vi "与工控机交互(子VI).vi"   [LabVIEW 2016, in "数据传输系统.lvlib"]
uses:
  <vilib>/ptbypt/NI_PtbyPt.lvlib
types:
  T1 = cluster{"setini":string, "sysini":string, "hechaini":string, "actualwrite":string, "actualread":string, "datasent":string, "反控命令信息队列":string, "反控与仪器交互":string}
  T2 = cluster{"仪器状态":u16[], "试剂余量":u16[], "各参数测量间隔":u16[], "关键参数":u16[], "校准点信息":u16[], "告警信息":u16[], "系统信息":u16[]}
  T3 = cluster{"[0]":bool, "[1]":bool, "[2]":bool, "[3]":bool, "[4]":bool}
  T4 = cluster{"[0]":bool, "[1]":bool, "[2]":bool, "[3]":bool, "[4]":bool, "[5]":bool}
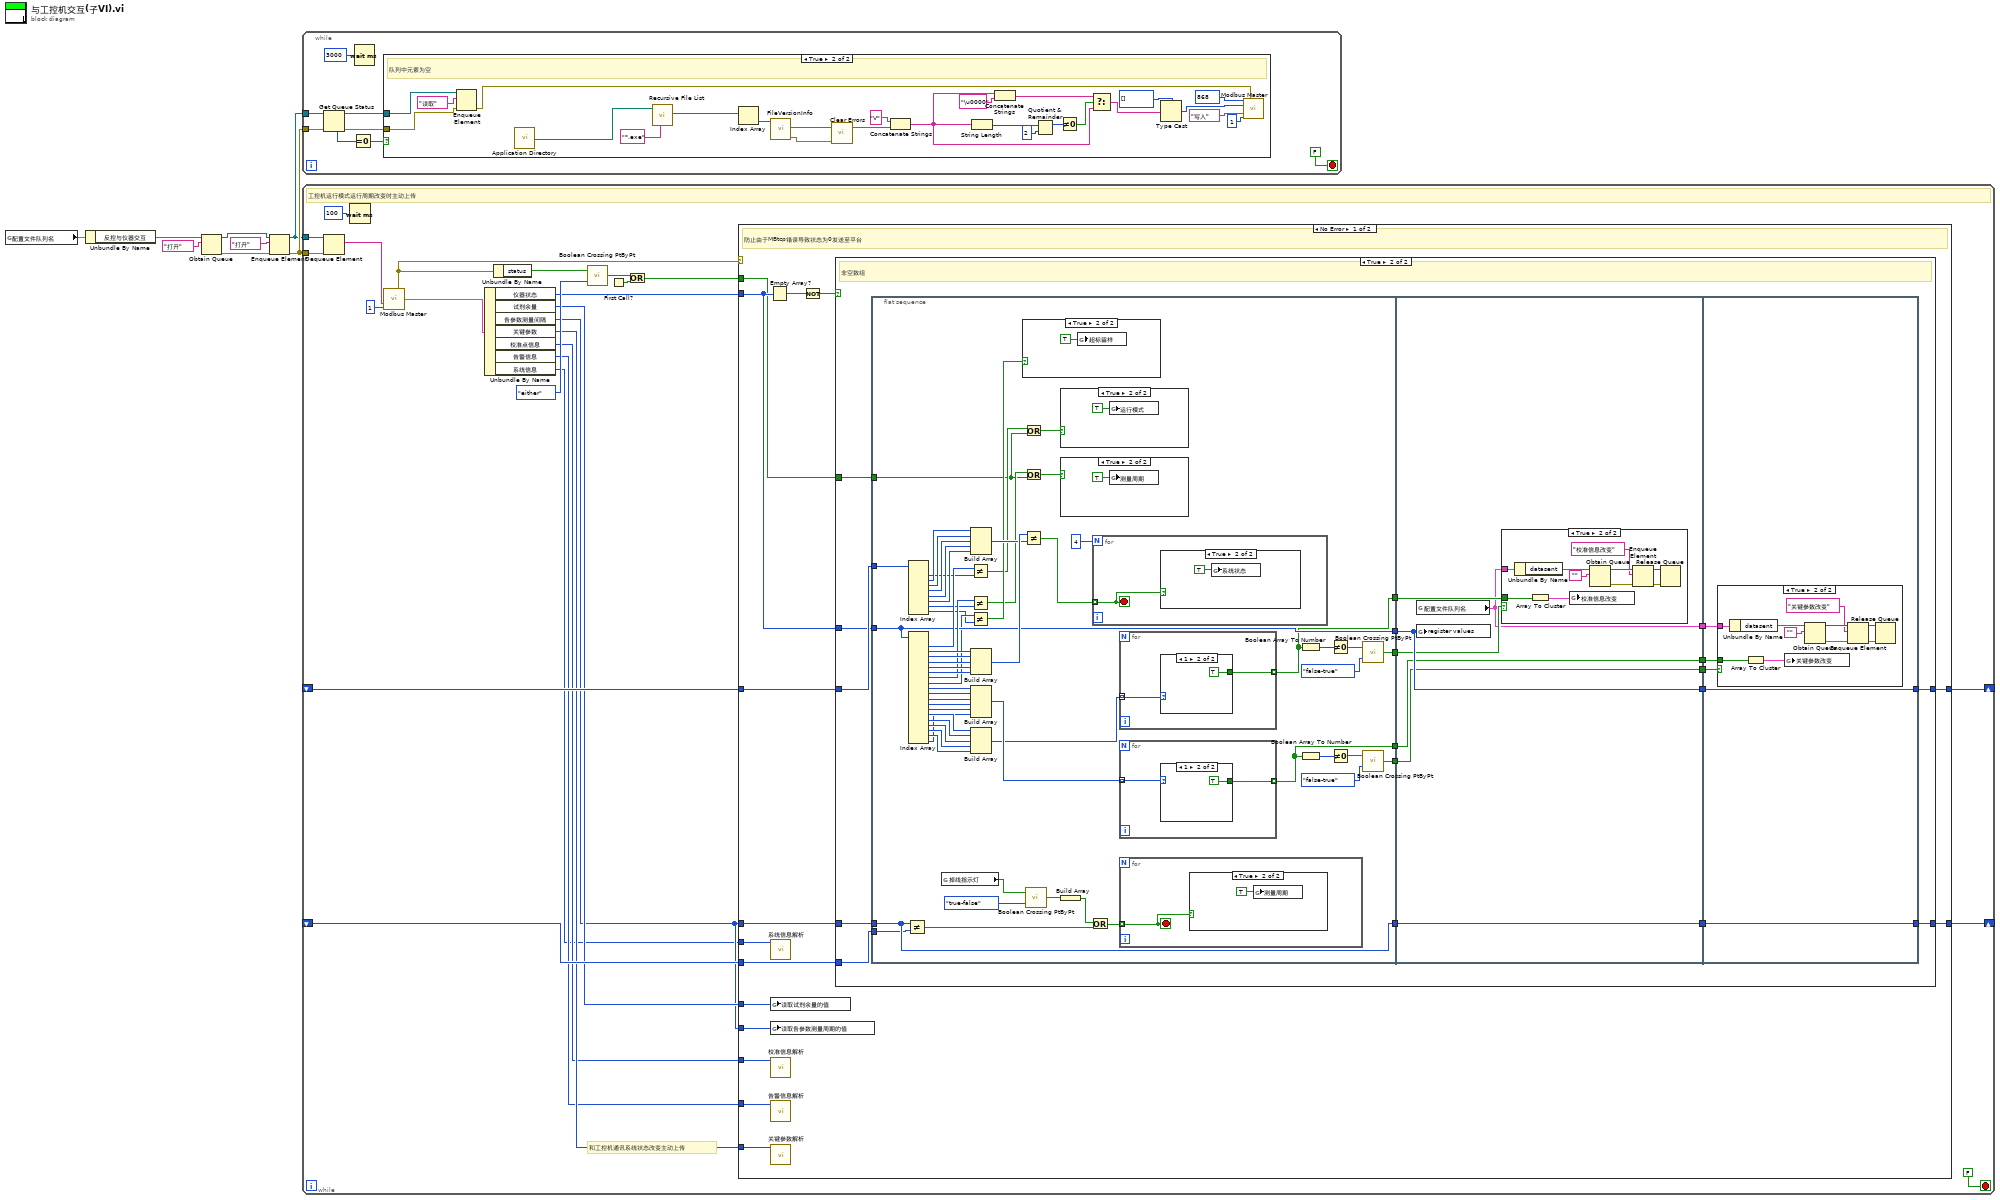
[diagram p0: block diagram]
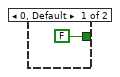
[diagram p4: hidden frame]
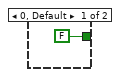
[diagram p5: hidden frame]
diagram:
  n1 = global read "全局1.vi" "配置文件队列名"() -> (w1:T1)
  n2 = Unbundle By Name(w1) -> ("反控与仪器交互"=w2:string)
  n3 = Obtain Queue(name (unnamed)=w2, element data type="打开" ("读取写入选择")) -> (queue out=w4:refnum<queue>, error out=w5:errorcluster)  [unwired: 3 in, 1 out]
  n4 = Enqueue Element(queue=w4, element="打开" ("读取写入选择"), error in (no error)=w5) -> (queue out=w6:refnum<queue>, error out=w7:errorcluster)  [unwired: 1 in, 1 out]
  n5 = while {
    tunnel: w6 -> [w13]
    tunnel: w7 -> [w12]
    stop <- FALSE stop-if-true
    n6 = Get Queue Status(queue=w13, error in (no error)=w12) -> (queue out=w10:refnum<queue>, error out=w9:errorcluster, # elements in queue=w14:i32)  [unwired: 1 in, 5 out]
    n7 = Equal To 0?(x=w14) -> (x = 0?=w11:bool)
    n8 = Wait (ms)(milliseconds to wait=u32 3000 ("等待时间（毫秒）")) -> ()  [unwired: 1 out]
    n9 = case shown="True" w11 {
      tunnel: w10 -> [_ w39]
      tunnel: w9 -> [_ w38]
      frame False {
      }
      frame True {
        # "队列中元素为空"
        n10 = Enqueue Element(queue=w39, element="读取" ("读取写入选择"), error in (no error)=w38) -> (error out=w34:errorcluster)  [unwired: 1 in, 2 out]
        n11 = call <vilib>:"Application Directory.vi"() -> ("Application Directory"=w32:path)
        n12 = call <vilib>:"Recursive File List.vi"("pattern"="*.exe", "Folder Path"=w32) -> ("All Files in Dir"=w30:path[])  [unwired: 5 in, 4 out]
        n13 = Index Array(array=w30) -> (element=w31:path)  [unwired: 1 in]
        n14 = call <vilib>:"FileVersionInfo.vi"("Application Path in"=w31) -> ("error out"=w17:errorcluster, "File Version Info"=w28:string)  [unwired: 7 in, 2 out]
        n15 = call <vilib>:"Clear Errors.vi"("error in (no error)"=w17) -> ()  [unwired: 5 in, 2 out]
        n16 = Concatenate Strings("V" ("字符串"), w28) -> (w20:string)
        n17 = String Length(string=w20) -> (length=w25:i32)
        n18 = Concatenate Strings(w20, "\u0000" ("字符串")) -> (w21:string)
        n19 = Quotient & Remainder(x=w25, y=2) -> (x-y*floor(x/y)=w23:i32)  [unwired: 1 out]
        n20 = Not Equal To 0?(x=w23) -> (x != 0?=w19:bool)
        n21 = Select(t=w21, s=w19, f=w20) -> (s? t:f=w18:string)
        n22 = Type Cast(type=u16[] [], x=w18) -> (*(type *) &x=w27:u16[])
        n23 = call "Modbus Master.vi"("starting address"=u16 868, "error in"=w34, "holding register values"=w27, "读取写入选择"="写入", "Unit ID"=u8 1) -> ()  [unwired: 4 in, 7 out]
      }
    }
  }
  n24 = while {
    tunnel: w6 -> [w61]
    tunnel: w7 -> [w60]
    shift-right: [w57] -> _
    shift-left: _ -> [w58]
    shift-right: [w50] -> _
    shift-left: _ -> [w49]
    stop <- FALSE stop-if-true
    # "和工控机通讯系统状态改变主动上传"
    # "工控机运行模式运行周期改变时主动上传"
    n25 = Dequeue Element(queue=w61, error in (no error)=w60) -> (element=w59:string)  [unwired: 1 in, 3 out]
    n26 = Wait (ms)(milliseconds to wait=u32 100 ("等待时间（毫秒）")) -> ()  [unwired: 1 out]
    n27 = call "Modbus Master.vi"("读取写入选择"=w59, "Unit ID"=u8 1) -> ("error out"=w56:errorcluster, "输出"=w48:T2)  [unwired: 7 in, 5 out]
    n28 = Unbundle By Name(w48) -> ("仪器状态"=w47:u16[], "试剂余量"=w46:u16[], "各参数测量间隔"=w45:u16[], "关键参数"=w44:u16[], "校准点信息"=w43:u16[], "告警信息"=w42:u16[], "系统信息"=w41:u16[])
    n29 = Unbundle By Name(w56) -> ("status"=w55:bool)
    n30 = call <vilib>:"Boolean Crossing PtByPt.vi"("direction"=enum16{"either", "false-true", "true-false"}."either", "input"=w55) -> ("crossing"=w53:bool)  [unwired: 1 in]
    n31 = First Call?() -> (First Call?: T/F=w52:bool)
    n32 = Or(x=w53, y=w52) -> (x .or. y?=w51:bool)
    n33 = case shown="No Error" w56 {
      tunnel: w47 -> [w77 _]
      tunnel: w58 -> [w79 w207]
      tunnel: [w78 w207] -> w57
      tunnel: w51 -> [w74 _]
      tunnel: w46 -> [w73 _]
      tunnel: w45 -> [w72 _]
      tunnel: w45 -> [w71 w206]
      tunnel: [w70 w206] -> w50
      tunnel: w49 -> [w69 _]
      tunnel: w44 -> [w68 _]
      tunnel: w43 -> [w67 _]
      tunnel: w42 -> [w66 _]
      tunnel: w41 -> [w65 _]
      frame No Error {
        # "防止由于MBtcp错误导致状态为0发送至平台"
        n34 = Empty Array?(array=w77) -> (empty?=w76:bool)
        n35 = call "系统信息解析.vi"("系统信息"=w65) -> ()  [unwired: 11 in]
        n36 = global write "全局1.vi" "读取试剂余量的值"(w73) -> ()
        n37 = global write "全局1.vi" "读取各参数测量周期的值"(w72) -> ()
        n38 = call "校准信息解析.vi"("校准信息"=w67) -> ()  [unwired: 11 in]
        n39 = call "告警信息解析.vi"("告警信息"=w66) -> ()  [unwired: 11 in]
        n40 = call "关键参数解析.vi"("关键参数"=w68) -> ()  [unwired: 11 in]
        n41 = Not(x=w76) -> (.not. x?=w75:bool)
        n42 = case shown="True" w75 {
          tunnel: w79 -> [w81 w98]
          tunnel: [w81 w97] -> w78
          tunnel: w77 -> [_ w96]
          tunnel: w74 -> [_ w95]
          tunnel: w71 -> [w80 w94]
          tunnel: [w80 w92] -> w70
          tunnel: w69 -> [_ w91]
          frame False {
          }
          frame True {
            # "非空数组"
            n43 = flat-sequence {
              tunnel: w96 -> [w142]
              tunnel: [w142] -> w99
              tunnel: w98 -> [w138]
              tunnel: w95 -> [w133]
              tunnel: w94 -> [w131]
              tunnel: [w131] -> w93
              tunnel: w91 -> [w130]
              tunnel: [w119] -> w90
              tunnel: [w108] -> w89
              tunnel: [w107] -> w88
              tunnel: [w106] -> w87
              tunnel: w99 -> [w180]
              tunnel: w93 -> [w179]
              tunnel: w90 -> [w175]
              tunnel: w89 -> [w178]
              tunnel: w88 -> [w177]
              tunnel: w87 -> [w176]
              tunnel: [w180] -> w86
              tunnel: [w179] -> w85
              tunnel: [w176] -> w84
              tunnel: [w175] -> w83
              tunnel: [w174] -> w82
              tunnel: [w194] -> w92
              tunnel: [w195] -> w97
              tunnel: w86 -> [w195]
              tunnel: w85 -> [w194]
              tunnel: w84 -> [w193]
              tunnel: w83 -> [w192]
              tunnel: w82 -> [w191]
              frame #0 {
                n44 = Not Equal?(x=w131, y=w130) -> (x != y?=w129:bool[])
                n45 = Index Array(array=w138) -> (element #1=w145:u16, element #2=w153:u16, element #3=w152:u16, element #4=w151:u16, element #5=w150:u16, element #6=w149:u16, element #7=w143:u16, element #8=w140:u16)  [unwired: 8 in]
                n46 = Index Array(array=w142) -> (element #1=w146:u16, element #2=w158:u16, element #3=w157:u16, element #4=w156:u16, element #5=w155:u16, element #6=w154:u16, element #7=w144:u16, element #8=w141:u16, element #9=w127:u16, element #10=w126:u16, element #11=w125:u16, element #12=w124:u16, element #13=w123:u16, element #14=w117:u16, element #15=w116:u16, element #16=w115:u16, element #17=w114:u16, element #18=w113:u16, element #19=w100:u16)  [unwired: 19 in]
                n47 = global read "全局 数据发送重叠.vi" "掉线指示灯"() -> (w104:bool)
                n48 = Not Equal?(x=w146, y=w145) -> (x != y?=w136:bool)
                n49 = Not Equal?(x=w144, y=w143) -> (x != y?=w134:bool)
                n50 = Not Equal?(x=w141, y=w140) -> (x != y?=w139:bool)
                n51 = Build Array(w153, w152, w151, w150, w149) -> (w147:u16[])
                n52 = Build Array(w158, w157, w156, w155, w154) -> (w148:u16[])
                n53 = Build Array(w127, w126, w125, w124, w123, w100) -> (w122:u16[])
                n54 = Build Array(w117, w116, w115, w114, w113) -> (w109:u16[])
                n55 = case shown="True" w139 {
                  frame False {
                  }
                  frame True {
                    n56 = global write "全局1.vi" "超标留样"(TRUE ("系统状态改变")) -> ()
                  }
                }
                n57 = Or(x=w136, y=w133) -> (x .or. y?=w135:bool)
                n58 = Or(x=w134, y=w133) -> (x .or. y?=w132:bool)
                n59 = Not Equal?(x=w148, y=w147) -> (x != y?=w137:bool[])
                n60 = call <vilib>:"Boolean Crossing PtByPt.vi"("direction"=enum16{"either", "false-true", "true-false"}."true-false", "input"=w104) -> ("crossing"=w102:bool)  [unwired: 1 in]
                n61 = case shown="True" w135 {
                  frame False {
                  }
                  frame True {
                    n62 = global write "全局1.vi" "运行模式"(TRUE) -> ()
                  }
                }
                n63 = case shown="True" w132 {
                  frame False {
                  }
                  frame True {
                    n64 = global write "全局1.vi" "测量周期"(TRUE ("系统状态改变")) -> ()
                  }
                }
                n65 = Build Array(w102) -> (w101:bool[])
                n66 = Or(x=w101, y=w129) -> (x .or. y?=w105:bool[])
                n67 = for {
                  N: 4 -> [_]
                  tunnel: w137 -> [w169] mode=indexing
                  stop <- w169 stop-if-true
                  n68 = case shown="True" w169 {
                    frame False {
                    }
                    frame True {
                      n69 = global write "全局1.vi" "系统状态"(TRUE ("系统状态改变")) -> ()
                    }
                  }
                }
                n70 = for {
                  tunnel: w109 -> [w160] mode=indexing
                  tunnel: [w159] -> w107 mode=indexing
                  n71 = case shown="1" w160 {
                    tunnel: [FALSE TRUE] -> w159
                    frame 0, Default {
                    }
                    frame 1 {
                    }
                  }
                }
                n72 = for {
                  tunnel: w122 -> [w164] mode=indexing
                  tunnel: [w163] -> w106 mode=indexing
                  n73 = case shown="1" w164 {
                    tunnel: [FALSE TRUE] -> w163
                    frame 0, Default {
                    }
                    frame 1 {
                    }
                  }
                }
                n74 = for {
                  tunnel: w105 -> [w167] mode=indexing
                  stop <- w167 stop-if-true
                  n75 = case shown="True" w167 {
                    frame False {
                    }
                    frame True {
                      n76 = global write "全局1.vi" "测量周期"(TRUE ("系统状态改变")) -> ()
                    }
                  }
                }
                n77 = Boolean Array To Number(Boolean array=w107) -> (number=w110:u32)
                n78 = Boolean Array To Number(Boolean array=w106) -> (number=w121:u32)
                n79 = Not Equal To 0?(x=w110) -> (x != 0?=w111:bool)
                n80 = Not Equal To 0?(x=w121) -> (x != 0?=w120:bool)
                n81 = call <vilib>:"Boolean Crossing PtByPt.vi"("direction"=enum16{"either", "false-true", "true-false"}."false-true", "input"=w111) -> ("crossing"=w108:bool)  [unwired: 1 in]
                n82 = call <vilib>:"Boolean Crossing PtByPt.vi"("direction"=enum16{"either", "false-true", "true-false"}."false-true", "input"=w120) -> ("crossing"=w119:bool)  [unwired: 1 in]
              }
              frame #1 {
                n83 = global read "全局1.vi" "配置文件队列名"() -> (w174:T1)
                n84 = global write "全局1.vi" "register values"(w180) -> ()
                n85 = case shown="True" w178 {
                  tunnel: w177 -> [_ w182]
                  tunnel: w174 -> [_ w181]
                  frame False {
                  }
                  frame True {
                    n86 = Unbundle By Name(w181) -> ("datasent"=w190:string)
                    n87 = Array To Cluster(array=w182) -> (cluster=w183:T3)
                    n88 = global write "全局1.vi" "校准信息改变"(w183) -> ()
                    n89 = Obtain Queue(name (unnamed)=w190, element data type="") -> (queue out=w188:refnum<queue>, error out=w186:errorcluster)  [unwired: 3 in, 1 out]
                    n90 = Enqueue Element(queue=w188, element="校准信息改变" ("元素"), error in (no error)=w186) -> (queue out=w185:refnum<queue>, error out=w184:errorcluster)  [unwired: 1 in, 1 out]
                    n91 = Release Queue(queue=w185, error in (no error)=w184) -> ()  [unwired: 1 in, 3 out]
                  }
                }
              }
              frame #2 {
                n92 = case shown="True" w192 {
                  tunnel: w193 -> [_ w197]
                  tunnel: w191 -> [_ w196]
                  frame False {
                  }
                  frame True {
                    n93 = Unbundle By Name(w196) -> ("datasent"=w205:string)
                    n94 = Array To Cluster(array=w197) -> (cluster=w198:T4)
                    n95 = global write "全局1.vi" "关键参数改变"(w198) -> ()
                    n96 = Obtain Queue(name (unnamed)=w205, element data type="") -> (queue out=w203:refnum<queue>, error out=w201:errorcluster)  [unwired: 3 in, 1 out]
                    n97 = Enqueue Element(queue=w203, element="关键参数改变" ("元素"), error in (no error)=w201) -> (queue out=w200:refnum<queue>, error out=w199:errorcluster)  [unwired: 1 in, 1 out]
                    n98 = Release Queue(queue=w200, error in (no error)=w199) -> ()  [unwired: 1 in, 3 out]
                  }
                }
              }
            }
          }
        }
      }
      frame Error {
      }
    }
  }
